vi "Utility - Geokon8001.vi"(8 "error in":errorcluster caption="错误输入（无错误）", 11 "VISA resource name":refnum<visa-resource-name>="COM2") -> (0 "error out":errorcluster caption="错误输出")   [LabVIEW 2015]
uses:
  <vilib>/Instr/_visa.llb/VISA Configure Serial Port (Instr).vi
panel:
  out "读取缓冲区":string
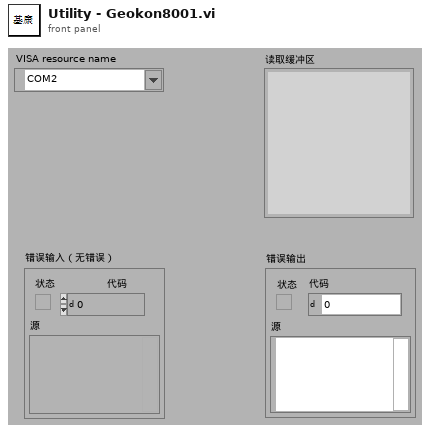
[diagram p1: front panel]
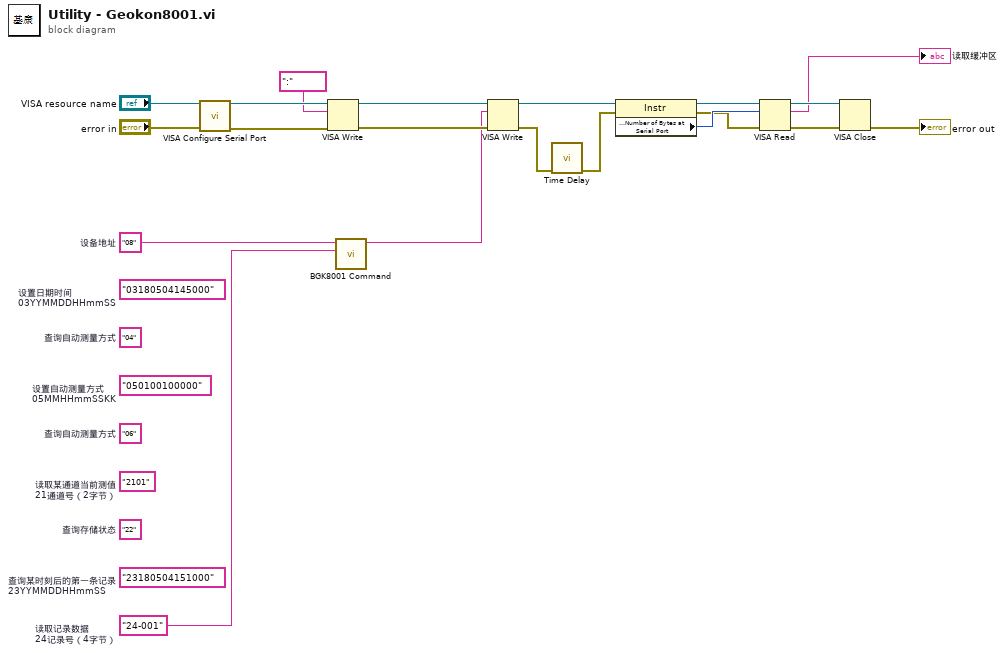
[diagram p0: block diagram]
diagram:
  (unwired) "04"  # 查询自动测量方式
  (unwired) "03180504145000"  # 设置日期时间 03YYMMDDHHmmSS
  w1 = "24-001"  # 读取记录数据 24记录号（4字节）
  (unwired) "23180504151000"  # 查询某时刻后的第一条记录 23YYMMDDHHmmSS
  (unwired) "22"  # 查询存储状态
  (unwired) "2101"  # 读取某通道当前测值 21通道号（2字节）
  (unwired) "06"  # 查询自动测量方式
  (unwired) "050100100000"  # 设置自动测量方式 05MMHHmmSSKK
  w2 = "08"  # 设备地址
  n1 = call-poly "VISA Configure Serial Port"("VISA resource name"="VISA resource name", "error in (no error)"="error in") -> ("VISA resource name out"=w18:refnum<visa-resource-name>, "error out"=w16:errorcluster)  [unwired: 12 in]
  n2 = VISA Write(VISA resource name=w18, write buffer=":" ("写入缓冲区"), error in (no error)=w16) -> (VISA resource name out=w17:refnum<visa-resource-name>, error out=w15:errorcluster)  [unwired: 1 out]
  n3 = call "BGK8001 Command.vi"("cmd code"=w1, "unit adress"=w2) -> ("cmd"=w4:string)  [unwired: 9 in]
  n4 = VISA Write(VISA resource name=w17, write buffer=w4, error in (no error)=w15) -> (VISA resource name out=w5:refnum<visa-resource-name>, error out=w8:errorcluster)  [unwired: 1 out]
  n5 = call "Time Delay"("error in (no error)"=w8) -> ("error out"=w7:errorcluster)  [unwired: 10 in]
  n6 = property class="Instr"(reference=w5, error in=w7) -> (reference out=w6:refnum<visa-resource-name>, error out=w11:errorcluster, "Serial Settings:Number of Bytes at Serial Port"=w12:u32)
  n7 = VISA Read(VISA resource name=w6, byte count=w12, error in (no error)=w11) -> (VISA resource name out=w10:refnum<visa-resource-name>, read buffer=→"读取缓冲区":string, error out=w9:errorcluster)  [unwired: 1 out]
  n8 = VISA Close(VISA resource name=w10, error in (no error)=w9) -> (error out=→"error out":errorcluster)
